vi "Z Slice.vi"() -> (0 "Z position":dbl)   [LabVIEW 2014]
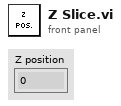
[diagram p1: front panel]
types:
  T1 = typedef "Image Acquisition Parameters.ctl" = cluster{"Scan Type":enum16{"Sample Scanning", "Beam Scanning"}, "Scan Mode":enum16{"XY", "XZ", "YZ", "XYZ"}, "Fast Axis Frequency (Hz)":dbl, "Image Format":u16, "Line Accumulations":u16, "Frames Per Capture":u16, "Frames Accumulations":u16, "Image Dimension (um)":dbl[], "Number of Z Steps":u8, "Z Steps Size (um)":dbl, "Pixel Size (nm)":dbl[], "Customized Image Format":dbl[]}
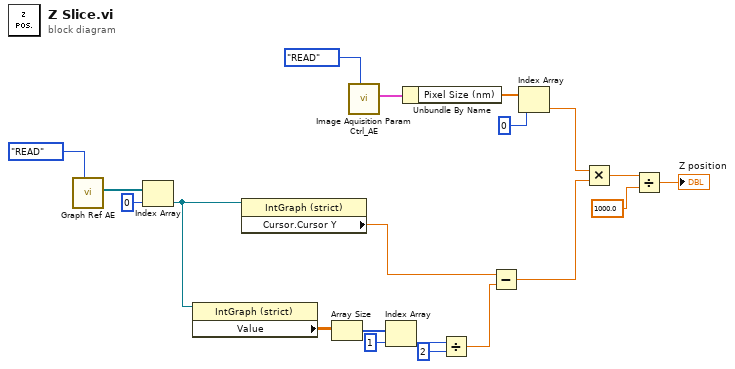
[diagram p0: block diagram]
diagram:
  n1 = call "Graph Ref AE.vi"("Action"=enum16{"READ", "WRITE"}."READ") -> ("Graph Ref Out"=w19:refnum<vi>[])  [unwired: 10 in]
  n2 = Index Array(array=w19, index=0) -> (element=w17:refnum<vi>)
  n3 = property class="IntGraph (strict)"(reference=w17) -> ("Value"=w16:sgl[][])  [unwired: 1 in, 2 out]
  n4 = property class="IntGraph (strict)"(reference=w17) -> ("Cursor.Cursor Y"=w1:dbl)  [unwired: 1 in, 2 out]
  n5 = Array Size(array=w16) -> (size(s)=w15:i32[])
  n6 = call "Image Aquisition Param Ctrl_AE.vi"("Action"=enum16{"READ", "WRITE"}."READ") -> ("Image Acquisition Parameters Out"=w10:T1)  [unwired: 10 in]
  n7 = Index Array(array=w15, index=1) -> (element=w13:i32)
  n8 = Unbundle By Name(w10) -> ("Pixel Size (nm)"=w9:dbl[])
  n9 = Divide(x=w13, y=2) -> (x/y=w2:dbl)
  n10 = Subtract(x=w1, y=w2) -> (x-y=w6:dbl)
  n11 = Index Array(array=w9, index=0) -> (element=w7:dbl)
  n12 = Multiply(x=w7, y=w6) -> (x*y=w4:dbl)
  n13 = Divide(x=w4, y=1000.0) -> (x/y=→"Z position":dbl)
